vi "Finish.vi"   [LabVIEW 2011]
doc: "This VI is called just before exiting. It is expected to close I/O refnum, save collected data, etc."
types:
  T1 = typedef "WPI_DigitalInputDevRef.ctl" = cluster{"DevStatus":errorcluster, "DIO Channel":T2, "Digital Module":T3}
  T2 = typedef "FPGA_DIOChannel.ctl" = enum8{"DIO 1", "DIO 2", "DIO 3", "DIO 4", "DIO 5", "DIO 6", "DIO 7", "DIO 8", "DIO 9", "DIO 10", "DIO 11", "DIO 12", "DIO 13", "DIO 14", "Invalid"}
  T3 = typedef "FPGA_TypedefDigitalModule.ctl" = enum16{"Digital Module 1", "Digital Module 2"}
  T4 = typedef "WPI_JoystickDevRef.ctl" = cluster{"Device":T5}
  T5 = typedef "WPI_JoystickDeviceEnum.ctl" = enum16{"USB 1", "USB 2", "USB 3", "USB 4", "Kinect 1", "Kinect 2"}
  T6 = typedef "WPI_MotorControlDeviceRef.ctl" = cluster{"DeviceStatus":errorcluster, "Type":enum16{"PWM", "CAN"}, "PWM":cluster{"Digital Module":T3, "PWM Channel":T7, "DeadBand":T8}, "CAN":cluster{"Device Number":u8, "Control Mode":T9, "Semaphore":T10, "Max Vout":dbl}, "Invert":bool, "TransformRef":T11, "InvTransformRef":T11}
  T7 = typedef "FPGA_DIOPWMChannel.ctl" = enum8{"PWM 1", "PWM 2", "PWM 3", "PWM 4", "PWM 5", "PWM 6", "PWM 7", "PWM 8", "PWM 9", "PWM 10", "Invalid"}
  T8 = typedef "WPI_PWMDeadband.ctl" = cluster{"Name":string, "maxPositivePwm":i32, "minPositivePwm":i32, "centerPwm":i32, "maxNegativePwm":i32, "minNegativePwm":i32, "angularRange":u16}
  T9 = typedef "WPI_CANJaguar_ControlMode.ctl" = enum8{"Percent VBus", "Current", "Speed", "Position", "Voltage"}
  T10 = typedef "Semaphore RefNum" = refnum<k1>
  T11 = typedef "WPI_PWMTransform_ConPane.ctl" = refnum<vi>
  T12 = typedef "WPI_I2CDevRef.ctl" = cluster{"DevStatus":errorcluster, "Digital Module":T3, "Device Address":u8}
  T13 = typedef "WPI_CounterDevRef.ctl" = cluster{"DevStatus":errorcluster, "CntIndex":T14}
  T14 = typedef "FPGA_CounterCtrSystemIndex.ctl" = enum8{"Ctr 0", "Ctr 1", "Ctr 2", "Ctr 3", "Ctr 4", "Ctr 5", "Ctr 6", "Ctr 7", "Invalid"}
  T15 = typedef "WPI_RobotDriveDevRef.ctl" = cluster{"DevStatus":errorcluster, "Motors[]":T6[], "Square Inputs":bool, "Max Output":dbl, "Isochronous":bool}
  T16 = typedef "WPI_CameraDevRef.ctl" = cluster{"Camera Address":string, "CameraStatus":errorcluster, "Acquire Image Notifier":refnum<notifier>}
  T17 = typedef "WPI_AnalogChannelDevRef.ctl" = cluster{"DevStatus":errorcluster, "Analog Module":T18, "Analog Channel":T19}
  T18 = typedef "FPGA_TypedefAnalogModule.ctl" = enum16{"Analog Module 1", "Analog Module 2"}
  T19 = typedef "FPGA_AIChannel.ctl" = enum8{"AI 1", "AI 2", "AI 3", "AI 4", "AI 5", "AI 6", "AI 7", "AI 8", "Invalid"}
  T20 = typedef "WPI_RelayDevRef.ctl" = cluster{"DevStatus":errorcluster, "Relay Channel":T21, "Digital Module":T3, "Relay Direction":T22}
  T21 = typedef "FPGA_DIORelayChannel.ctl" = enum8{"Relay 1", "Relay 2", "Relay 3", "Relay 4", "Relay 5", "Relay 6", "Relay 7", "Relay 8", "Invalid"}
  T22 = typedef "WPI_RelayDirection.ctl" = enum16{"Both directions", "Forward only", "Reverse only"}
  T23 = typedef "WPI_GyroDevRef.ctl" = cluster{"DevStatus":errorcluster, "Analog Module":T18, "Analog Channel":T19, "Offset":dbl, "Gain (VoltsPerDegree/Second)":dbl}
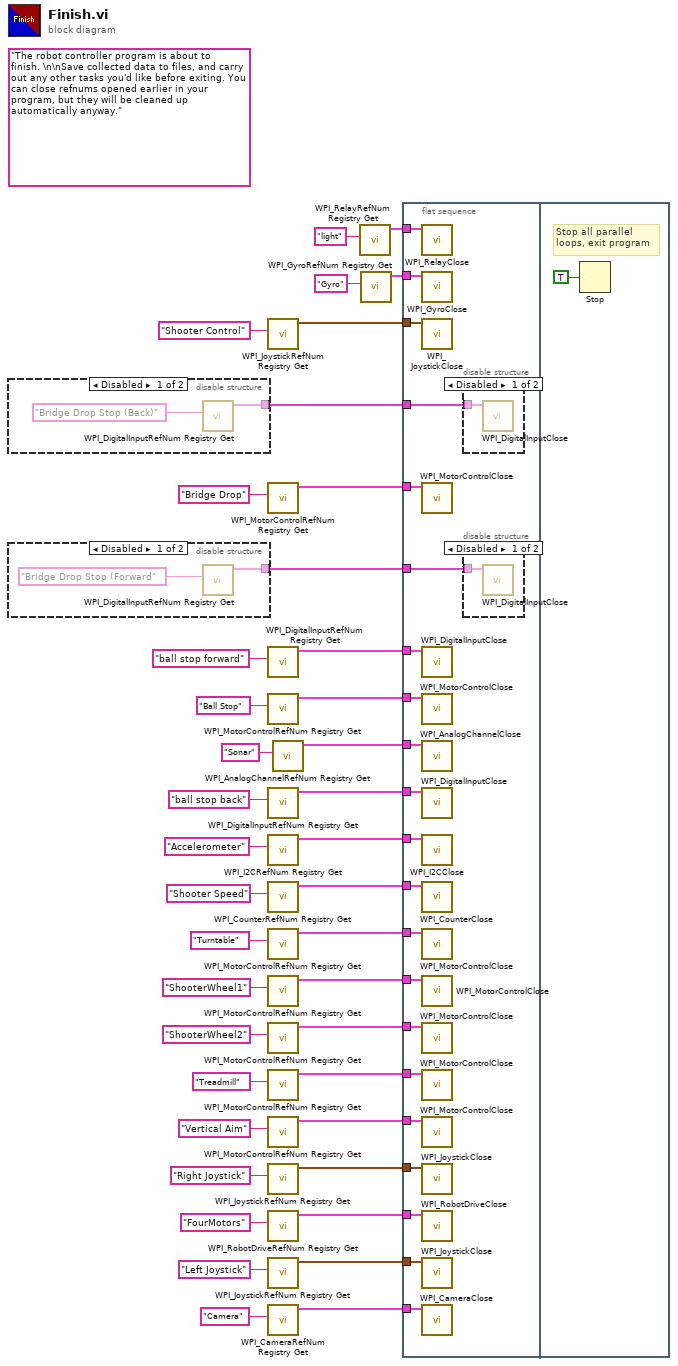
[diagram p0: block diagram]
diagram:
  (unwired) "The robot controller program is about to finish. \n\nSave collected data to files, and carry out any other tasks you'd like before exiting. You can close refnums opened earlier in your program, but they will be cleaned up automatically anyway."
  n1 = disable-structure shown="Disabled" {
    disable-tunnel: [w42 _] -> w9
    frame Disabled {
      n2 = call <vilib>:"WPI_DigitalInputRefNum Registry Get.vi"("refnum name"="Bridge Drop Stop (Back)") -> ("DigitalInputDevRef"=w42:T1)  [unwired: 9 in, 1 out]
    }
    frame Enabled {
    }
  }
  n3 = disable-structure shown="Disabled" {
    disable-tunnel: [w44 _] -> w8
    frame Disabled {
      n4 = call <vilib>:"WPI_DigitalInputRefNum Registry Get.vi"("refnum name"="Bridge Drop Stop (Forward") -> ("DigitalInputDevRef"=w44:T1)  [unwired: 9 in, 1 out]
    }
    frame Enabled {
    }
  }
  n5 = call <vilib>:"WPI_JoystickRefNum Registry Get.vi"("refnum name"="Shooter Control") -> ("JoystickDevRef"=w32:T4)  [unwired: 9 in, 1 out]
  n6 = call <vilib>:"WPI_MotorControlRefNum Registry Get.vi"("refnum name"="Bridge Drop") -> ("MotorControlDevRef"=w10:T6)  [unwired: 9 in, 1 out]
  n7 = call <vilib>:"WPI_DigitalInputRefNum Registry Get.vi"("refnum name"="ball stop forward") -> ("DigitalInputDevRef"=w2:T1)  [unwired: 9 in, 1 out]
  n8 = call <vilib>:"WPI_MotorControlRefNum Registry Get.vi"("refnum name"="Ball Stop") -> ("MotorControlDevRef"=w20:T6)  [unwired: 9 in, 1 out]
  n9 = call <vilib>:"WPI_DigitalInputRefNum Registry Get.vi"("refnum name"="ball stop back") -> ("DigitalInputDevRef"=w4:T1)  [unwired: 9 in, 1 out]
  n10 = call <vilib>:"WPI_I2CRefNum Registry Get.vi"("refnum name"="Accelerometer") -> ("I2CDevRef"=w12:T12)  [unwired: 9 in, 1 out]
  n11 = call <vilib>:"WPI_CounterRefNum Registry Get.vi"("refnum name"="Shooter Speed") -> ("CounterDevRef"=w16:T13)  [unwired: 9 in, 1 out]
  n12 = call <vilib>:"WPI_MotorControlRefNum Registry Get.vi"("refnum name"="Turntable") -> ("MotorControlDevRef"=w22:T6)  [unwired: 9 in, 1 out]
  n13 = call <vilib>:"WPI_MotorControlRefNum Registry Get.vi"("refnum name"="ShooterWheel1") -> ("MotorControlDevRef"=w26:T6)  [unwired: 9 in, 1 out]
  n14 = call <vilib>:"WPI_MotorControlRefNum Registry Get.vi"("refnum name"="ShooterWheel2") -> ("MotorControlDevRef"=w24:T6)  [unwired: 9 in, 1 out]
  n15 = call <vilib>:"WPI_MotorControlRefNum Registry Get.vi"("refnum name"="Treadmill") -> ("MotorControlDevRef"=w28:T6)  [unwired: 9 in, 1 out]
  n16 = call <vilib>:"WPI_MotorControlRefNum Registry Get.vi"("refnum name"="Vertical Aim") -> ("MotorControlDevRef"=w30:T6)  [unwired: 9 in, 1 out]
  n17 = call <vilib>:"WPI_JoystickRefNum Registry Get.vi"("refnum name"="Right Joystick") -> ("JoystickDevRef"=w37:T4)  [unwired: 1 in, 9 out]
  n18 = call <vilib>:"WPI_RobotDriveRefNum Registry Get.vi"("refnum name"="FourMotors") -> ("RobotDriveDevRef"=w38:T15)  [unwired: 1 in, 9 out]
  n19 = call <vilib>:"WPI_JoystickRefNum Registry Get.vi"("refnum name"="Left Joystick") -> ("JoystickDevRef"=w33:T4)  [unwired: 9 in, 1 out]
  n20 = call <vilib>:"WPI_CameraRefNum Registry Get.vi"("refnum name"="Camera") -> ("CameraDevRef"=w36:T16)  [unwired: 1 in, 9 out]
  n21 = call <vilib>:"WPI_AnalogChannelRefNum Registry Get.vi"("refnum name"="Sonar") -> ("AIDeviceRef"=w18:T17)  [unwired: 9 in, 1 out]
  n22 = call <vilib>:"WPI_RelayRefNum Registry Get.vi"("refnum name"="light") -> ("RelayDevRef"=w6:T20)  [unwired: 9 in, 1 out]
  n23 = call <vilib>:"WPI_GyroRefNum Registry Get.vi"("refnum name"="Gyro") -> ("GyroDevRef"=w14:T23)  [unwired: 9 in, 1 out]
  n24 = flat-sequence {
    tunnel: w38 -> [w65]
    tunnel: w37 -> [w64]
    tunnel: w36 -> [w63]
    tunnel: w33 -> [w62]
    tunnel: w32 -> [w61]
    tunnel: w30 -> [w60]
    tunnel: w28 -> [w59]
    tunnel: w24 -> [w58]
    tunnel: w26 -> [w57]
    tunnel: w22 -> [w56]
    tunnel: w20 -> [w55]
    tunnel: w18 -> [w54]
    tunnel: w16 -> [w53]
    tunnel: w14 -> [w52]
    tunnel: w12 -> [w51]
    tunnel: w10 -> [w50]
    tunnel: w9 -> [w49]
    tunnel: w8 -> [w48]
    tunnel: w6 -> [w47]
    tunnel: w4 -> [w46]
    tunnel: w2 -> [w45]
    frame #0 {
      n25 = call <vilib>:"WPI_RelayClose.vi"("RelayDevRef"=w47) -> ()  [unwired: 10 in, 1 out]
      n26 = call <vilib>:"WPI_GyroClose.vi"("GyroDevRef"=w52) -> ()  [unwired: 1 in, 10 out]
      n27 = call <vilib>:"WPI_JoystickClose.vi"("JoystickDevRef"=w61) -> ()  [unwired: 11 in]
      n28 = call <vilib>:"WPI_MotorControlClose.vi"("MotorControlDevRef"=w50) -> ()  [unwired: 10 in, 1 out]
      n29 = call <vilib>:"WPI_DigitalInputClose.vi"("DigitalInputDevRef"=w45) -> ()  [unwired: 10 in, 1 out]
      n30 = call <vilib>:"WPI_MotorControlClose.vi"("MotorControlDevRef"=w55) -> ()  [unwired: 10 in, 1 out]
      n31 = call <vilib>:"WPI_AnalogChannelClose.vi"("AIDeviceRef"=w54) -> ()  [unwired: 10 in, 1 out]
      n32 = call <vilib>:"WPI_DigitalInputClose.vi"("DigitalInputDevRef"=w46) -> ()  [unwired: 10 in, 1 out]
      n33 = call <vilib>:"WPI_I2CClose.vi"("I2CDevRef"=w51) -> ()  [unwired: 1 in, 10 out]
      n34 = call <vilib>:"WPI_CounterClose.vi"("CounterDevRef"=w53) -> ()  [unwired: 10 in, 1 out]
      n35 = call <vilib>:"WPI_MotorControlClose.vi"("MotorControlDevRef"=w56) -> ()  [unwired: 10 in, 1 out]
      n36 = call <vilib>:"WPI_MotorControlClose.vi"("MotorControlDevRef"=w57) -> ()  [unwired: 10 in, 1 out]
      n37 = call <vilib>:"WPI_MotorControlClose.vi"("MotorControlDevRef"=w58) -> ()  [unwired: 10 in, 1 out]
      n38 = call <vilib>:"WPI_MotorControlClose.vi"("MotorControlDevRef"=w59) -> ()  [unwired: 10 in, 1 out]
      n39 = call <vilib>:"WPI_MotorControlClose.vi"("MotorControlDevRef"=w60) -> ()  [unwired: 10 in, 1 out]
      n40 = call <vilib>:"WPI_JoystickClose.vi"("JoystickDevRef"=w64) -> ()  [unwired: 11 out]
      n41 = call <vilib>:"WPI_RobotDriveClose.vi"("RobotDriveDevRef"=w65) -> ()  [unwired: 1 in, 10 out]
      n42 = call <vilib>:"WPI_JoystickClose.vi"("JoystickDevRef"=w62) -> ()  [unwired: 11 in]
      n43 = call <vilib>:"WPI_CameraClose.vi"("CameraDevRef"=w63) -> ()  [unwired: 1 in, 10 out]
      n44 = disable-structure shown="Disabled" {
        disable-tunnel: w49 -> [w66 _]
        frame Disabled {
          n45 = call <vilib>:"WPI_DigitalInputClose.vi"("DigitalInputDevRef"=w66) -> ()  [unwired: 10 in, 1 out]
        }
        frame Enabled {
        }
      }
      n46 = disable-structure shown="Disabled" {
        disable-tunnel: w48 -> [w67 _]
        frame Disabled {
          n47 = call <vilib>:"WPI_DigitalInputClose.vi"("DigitalInputDevRef"=w67) -> ()  [unwired: 10 in, 1 out]
        }
        frame Enabled {
        }
      }
    }
    frame #1 {
      # "Stop all parallel\nloops, exit program"
      n48 = Stop(stop? (T)=TRUE ("Quit")) -> ()
    }
  }
